vi "extract_wavelength.vi"(0 "Path_image":path=path "C:/Users/swift/Desktop/Python/imec/Data/SKFX.300x300.Binning.2.frame.1.Gain.1.time.5.HDR-V6_corrected.hdr") -> (1 "WAVELENGTH":sgl[](array[numeric]), 2 "WAVELENGTH NUMBER":i32)   [LabVIEW 2018]
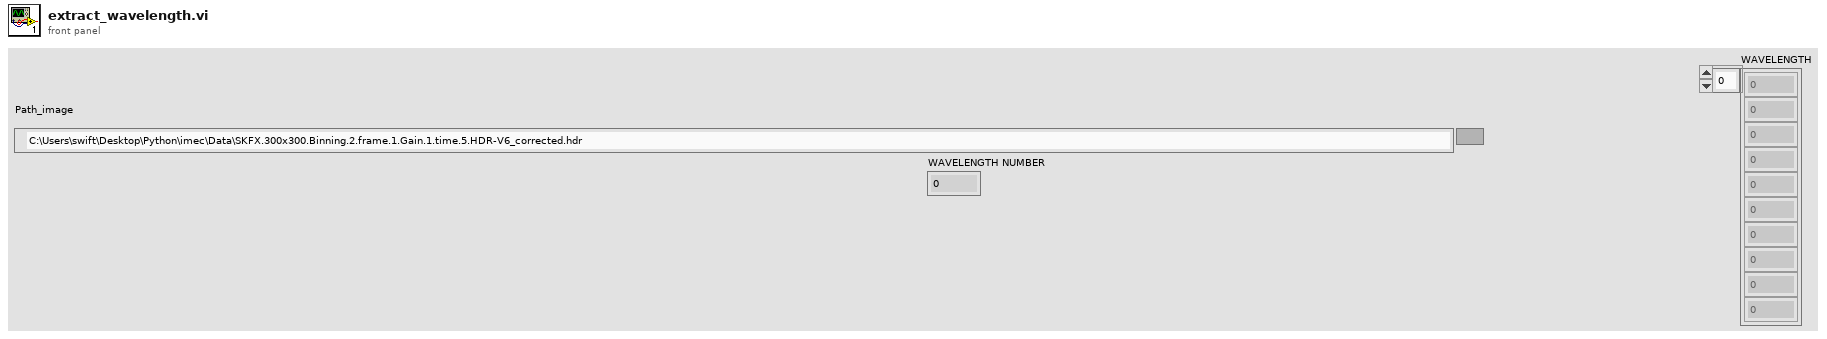
[diagram p1: front panel]
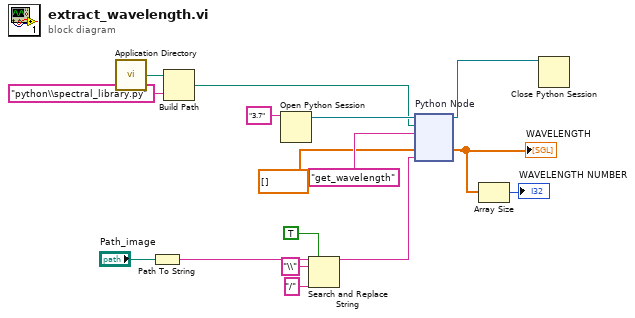
[diagram p0: block diagram]
diagram:
  n1 = call <vilib>:"Application Directory.vi"() -> ("Application Directory"=w4:path)
  n2 = Path To String(path="Path_image") -> (string=w15:string)
  n3 = Build Path(base path=w4, name or relative path="python\\spectral_library.py" ("nom ou chemin relatif")) -> (appended path=w2:path)
  n4 = Open Python Session(python version="3.7" ("Python version")) -> (session out=w10:refnum<k35>)  [unwired: 2 in, 1 out]
  n5 = Search and Replace String(replace all?=TRUE ("replace all? (F)"), input string=w15, search string="\\", replace string="/" ("replace string (\"\")")) -> (result string=w7:string)  [unwired: 4 in, 3 out]
  n6 = node "Python Node"(w10, w2, "get_wavelength" ("function name"), sgl[] [], w7) -> (w1:refnum<k35>, w6:sgl[])  [unwired: 2 in, 3 out]
  "WAVELENGTH" <- w6
  n7 = Array Size(array=w6) -> (size(s)=→"WAVELENGTH NUMBER":i32)
  n8 = Close Python Session(session in=w1) -> ()  [unwired: 1 in, 1 out]
